vi "Untitled 2.vi"() -> ()   [LabVIEW 2017, in "SQLite.lvclass"]
uses:
  SQLite.lvclass
  <userlib>/sushu/sushu.lvlib
panel:
  out "String 2":string
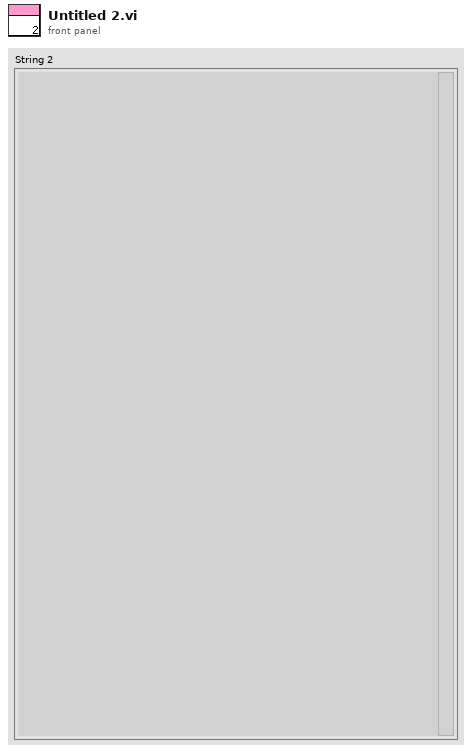
[diagram p1: front panel]
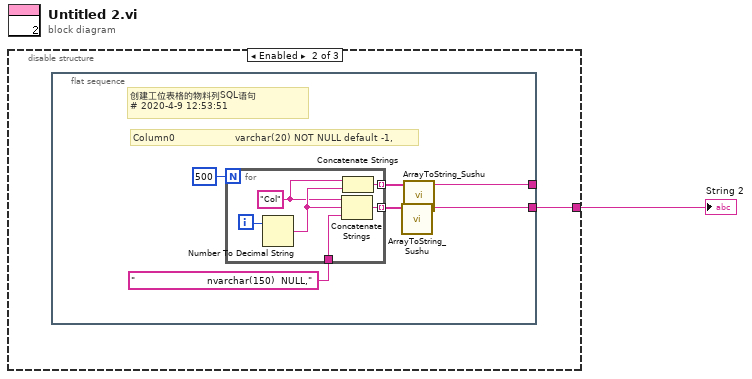
[diagram p0: block diagram]
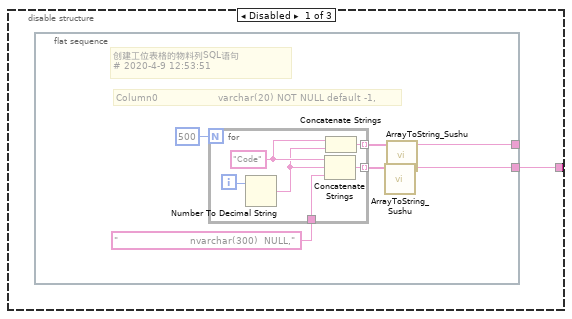
[diagram p2: hidden frame]
diagram:
  n1 = disable-structure shown="Enabled" {
    disable-tunnel: [w2 w15 _] -> w1
    frame Disabled {
      n2 = flat-sequence {
        tunnel: [w6] -> w2
        tunnel: [w4] -> _
        frame #0 {
          # "创建工位表格的物料列SQL语句\n# 2020-4-9 12:53:51"
          # "Column0                    varchar(20) NOT NULL default -1,"
          n3 = for {
            N: 500 -> [_]
            tunnel: [w13] -> w7 mode=indexing
            tunnel: "                        nvarchar(300)  NULL," ("string") -> [w12]
            tunnel: [w9] -> w5 mode=indexing
            i -> [w14]
            w11 = "Code" ("string")
            n4 = Number To Decimal String(number=w14) -> (decimal integer string=w10:string)  [unwired: 1 in]
            n5 = Concatenate Strings(w11, w10, w12) -> (w13:string)
            n6 = Concatenate Strings(w11, w10) -> (w9:string)
          }
          n7 = call <userlib>:"ArrayToString_Sushu.vi"("Array"=w7) -> ("String"=w6:string)  [unwired: 10 in]
          n8 = call <userlib>:"ArrayToString_Sushu.vi"("Array"=w5) -> ("String"=w4:string)  [unwired: 10 in]
        }
      }
    }
    frame Enabled {
      n9 = flat-sequence {
        tunnel: [w19] -> w15
        tunnel: [w17] -> _
        frame #0 {
          # "创建工位表格的物料列SQL语句\n# 2020-4-9 12:53:51"
          # "Column0                    varchar(20) NOT NULL default -1,"
          n10 = for {
            N: 500 -> [_]
            tunnel: [w26] -> w20 mode=indexing
            tunnel: "                        nvarchar(150)  NULL," ("string") -> [w25]
            tunnel: [w23] -> w18 mode=indexing
            i -> [w27]
            w22 = "Col" ("string")
            n11 = Number To Decimal String(number=w27) -> (decimal integer string=w24:string)  [unwired: 1 in]
            n12 = Concatenate Strings(w22, w24, w25) -> (w26:string)
            n13 = Concatenate Strings(w22, w24) -> (w23:string)
          }
          n14 = call <userlib>:"ArrayToString_Sushu.vi"("Array"=w20) -> ("String"=w19:string)  [unwired: 10 in]
          n15 = call <userlib>:"ArrayToString_Sushu.vi"("Array"=w18) -> ("String"=w17:string)  [unwired: 10 in]
        }
      }
    }
    frame Disabled {
    }
  }
  "String 2" <- w1
